vi "Panel Event.vi"(10 "Events":T1, 11 "Panel Event in":refnum<class "Panel Event.lvclass">) -> (0 "error out":errorcluster, 3 "Panel Event out":refnum<class "Panel Event.lvclass">)   [LabVIEW 2021, in "Panel Event.lvlib" / "Panel Event.lvclass"]
uses:
  Panel Event.lvclass
  Events.ctl
  Panel Event.lvlib
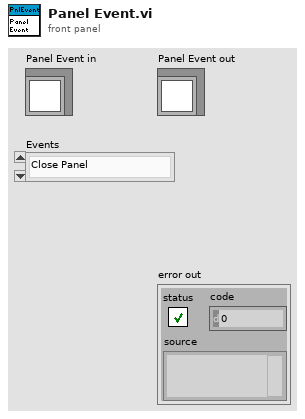
[diagram p1: front panel]
types:
  T1 = typedef "Panel Event.lvlib/Events.ctl" = enum16{"Close Panel", "Show Panel", "Hide Panel"}
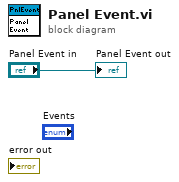
[diagram p0: block diagram]
diagram:
  "Panel Event out" <- "Panel Event in"
